vi "New Input Gallery.vi"(8 "Error In":errorcluster) -> (0 "Error Out":errorcluster, 3 "New Input Gallery":refnum<class "QWidget.lvclass">)   [LabVIEW 2014]
doc: "Dynamically assembles a widget that contains a variety of input widgets (text editors, combo boxes, and spinboxes). These widgets are grouped within group boxes.\n\nThe caller must manually make the returned widget visible.\n\n\nCopyright (c) 2019 Sze Howe Koh.\nThis code is licensed under the MIT license."
uses:
  <vilib>/addons/LQ/Qt Widgets/QWidget/QWidget.lvclass
  <vilib>/addons/LQ/Qt Widgets/QBoxLayout/Direction.ctl
  <vilib>/addons/LQ/Qt Widgets/QLineEdit/EchoMode.ctl
  <vilib>/addons/LQ/Qt Widgets/QLineEdit/setPlaceholderText.vi
  <vilib>/addons/LQ/Qt Widgets/QLineEdit/setEchoMode.vi
  <vilib>/addons/LQ/Qt Widgets/QTextEdit/QTextEdit.lvclass
  <vilib>/addons/LQ/Qt Widgets/QLineEdit/QLineEdit.lvclass
  <vilib>/addons/LQ/Qt Widgets/QGroupBox/QGroupBox.lvclass
  <vilib>/addons/LQ/Qt Widgets/QBoxLayout/QBoxLayout.lvclass
  <vilib>/addons/LQ/Qt Widgets/QComboBox/QComboBox.lvclass
  <vilib>/addons/LQ/Qt Widgets/QSpinBox/QSpinBox.lvclass
  <vilib>/addons/LQ/Qt Widgets/QDoubleSpinBox/QDoubleSpinBox.lvclass
  <vilib>/addons/LQ/Qt Widgets/QFontComboBox/QFontComboBox.lvclass
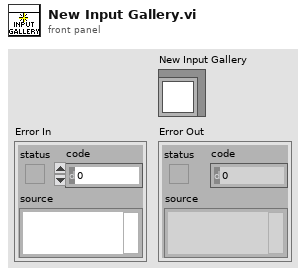
[diagram p1: front panel]
types:
  T1 = typedef "QLineEdit.lvclass/EchoMode.ctl" = i32
  T2 = typedef "QBoxLayout.lvclass/Direction.ctl" = i32
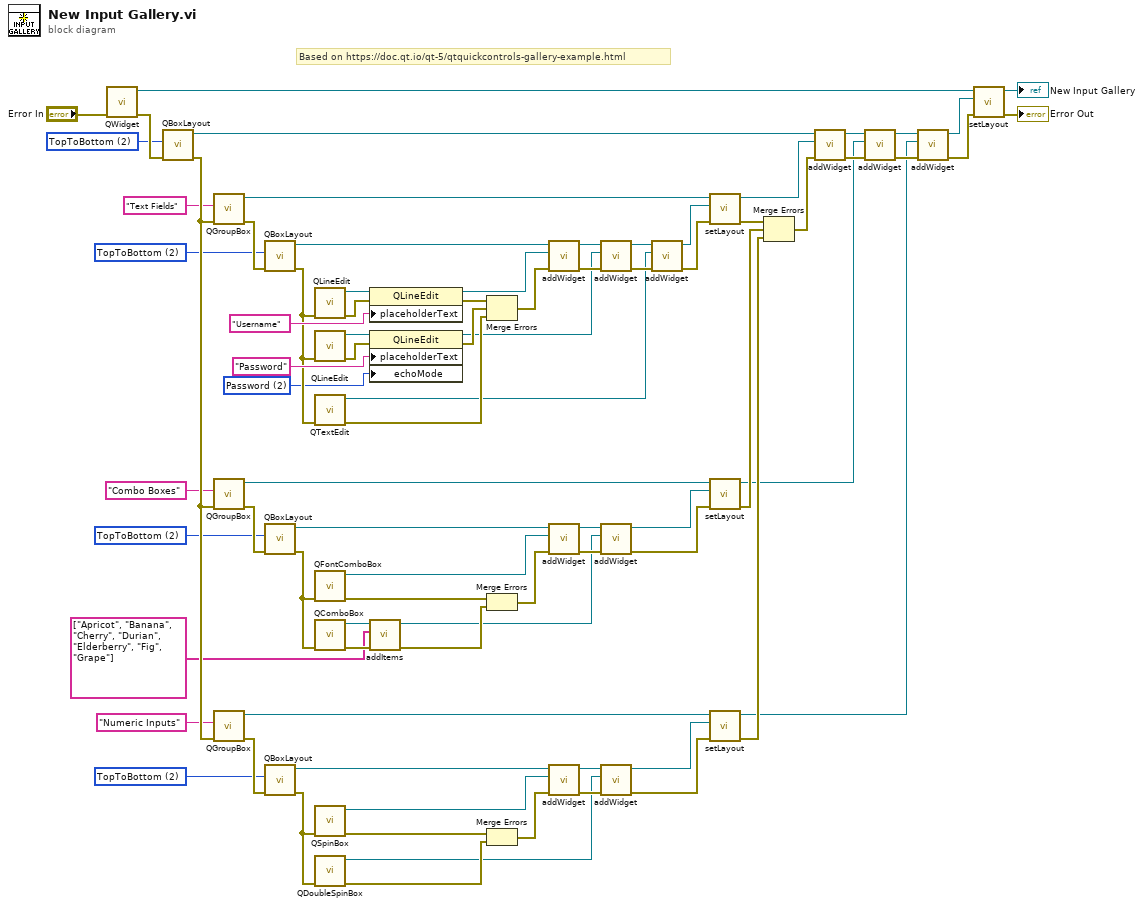
[diagram p0: block diagram]
diagram:
  w8 = T1 2 items=["Normal", "NoEcho", "Password", "PasswordEchoOnEdit"] ("echoMode")
  w48 = T2 2 items=["LeftToRight", "RightToLeft", "TopToBottom", "BottomToTop"] ("direction")
  w55 = T2 2 items=["LeftToRight", "RightToLeft", "TopToBottom", "BottomToTop"] ("direction")
  w56 = T2 2 items=["LeftToRight", "RightToLeft", "TopToBottom", "BottomToTop"] ("direction")
  w57 = T2 2 items=["LeftToRight", "RightToLeft", "TopToBottom", "BottomToTop"] ("direction")
  # "Based on https://doc.qt.io/qt-5/qtquickcontrols-gallery-example.html"
  n1 = call <vilib>:"QWidget.vi"("Error In"="Error In") -> ("Error Out"=w77:errorcluster, "New QWidget"=w58:refnum<class "QWidget.lvclass">)  [unwired: 9 in]
  n2 = call <vilib>:"QBoxLayout.vi"("Error In"=w77, "direction"=w56) -> ("Error Out"=w72:errorcluster, "New QBoxLayout"=w60:refnum<class "QBoxLayout.lvclass">)  [unwired: 8 in]
  n3 = call <vilib>:"QGroupBox.vi"("Error In"=w72, "title"="Text Fields") -> ("Error Out"=w78:errorcluster, "New QGroupBox"=w68:refnum<class "QGroupBox.lvclass">)  [unwired: 8 in]
  n4 = call <vilib>:"QGroupBox.vi"("Error In"=w72, "title"="Combo Boxes") -> ("Error Out"=w74:errorcluster, "New QGroupBox"=w61:refnum<class "QGroupBox.lvclass">)  [unwired: 8 in]
  n5 = call <vilib>:"QGroupBox.vi"("Error In"=w72, "title"="Numeric Inputs") -> ("Error Out"=w71:errorcluster, "New QGroupBox"=w41:refnum<class "QGroupBox.lvclass">)  [unwired: 8 in]
  n6 = call <vilib>:"QBoxLayout.vi"("Error In"=w78, "direction"=w57) -> ("Error Out"=w14:errorcluster, "New QBoxLayout"=w67:refnum<class "QBoxLayout.lvclass">)  [unwired: 8 in]
  n7 = call <vilib>:"QBoxLayout.vi"("Error In"=w74, "direction"=w55) -> ("Error Out"=w73:errorcluster, "New QBoxLayout"=w63:refnum<class "QBoxLayout.lvclass">)  [unwired: 8 in]
  n8 = call <vilib>:"QBoxLayout.vi"("Error In"=w71, "direction"=w48) -> ("Error Out"=w70:errorcluster, "New QBoxLayout"=w46:refnum<class "QBoxLayout.lvclass">)  [unwired: 8 in]
  n9 = call <vilib>:"QLineEdit.vi"("Error In"=w14) -> ("Error Out"=w18:errorcluster, "New QLineEdit"=w20:refnum<class "QLineEdit.lvclass">)  [unwired: 9 in]
  n10 = call <vilib>:"QLineEdit.vi"("Error In"=w14) -> ("Error Out"=w21:errorcluster, "New QLineEdit"=w23:refnum<class "QLineEdit.lvclass">)  [unwired: 9 in]
  n11 = call <vilib>:"QTextEdit.vi"("Error In"=w14) -> ("Error Out"=w80:errorcluster, "New QTextEdit"=w9:refnum<class "QTextEdit.lvclass">)  [unwired: 9 in]
  n12 = call <vilib>:"QFontComboBox.vi"("Error In"=w73) -> ("Error Out"=w53:errorcluster, "New QFontComboBox"=w26:refnum<class "QFontComboBox.lvclass">)  [unwired: 9 in]
  n13 = call <vilib>:"QComboBox.vi"("Error In"=w73) -> ("Error Out"=w4:errorcluster, "New QComboBox"=w5:refnum<class "QComboBox.lvclass">)  [unwired: 9 in]
  n14 = call <vilib>:"QSpinBox.vi"("Error In"=w70) -> ("Error Out"=w45:errorcluster, "New QSpinBox"=w28:refnum<class "QSpinBox.lvclass">)  [unwired: 9 in]
  n15 = call <vilib>:"QDoubleSpinBox.vi"("Error In"=w70) -> ("Error Out"=w44:errorcluster, "New QDoubleSpinBox"=w27:refnum<class "QDoubleSpinBox.lvclass">)  [unwired: 9 in]
  n16 = property class="QLineEdit"(reference=w20, error in=w18, "placeholderText"="Username" ("text")) -> (reference out=w19:refnum<class "QLineEdit.lvclass">, error out=w17:errorcluster)
  n17 = property class="QLineEdit"(reference=w23, error in=w21, "placeholderText"="Password" ("text"), "echoMode"=w8) -> (reference out=w22:refnum<class "QLineEdit.lvclass">, error out=w79:errorcluster)
  n18 = call <vilib>:"addItems.vi"("Error In"=w4, "texts"=string[] ["Apricot", "Banana", "Cherry", "Durian", "Elderberry", "Fig", "Grape"], "QComboBox In"=w5) -> ("Error Out"=w3:errorcluster, "QComboBox Out"=w2:refnum<class "QComboBox.lvclass">)  [unwired: 7 in]
  n19 = Merge Errors(w17, w79, w80) -> (w54:errorcluster)
  n20 = Merge Errors(w53, w3) -> (w52:errorcluster)
  n21 = Merge Errors(w45, w44) -> (w43:errorcluster)
  n22 = call <vilib>:"addWidget.vi"("Error In"=w54, "widget"=w19, "QBoxLayout In"=w67) -> ("Error Out"=w76:errorcluster, "QBoxLayout Out"=w66:refnum<class "QBoxLayout.lvclass">)  [unwired: 7 in]
  n23 = call <vilib>:"addWidget.vi"("Error In"=w52, "widget"=w26, "QBoxLayout In"=w63) -> ("Error Out"=w75:errorcluster, "QBoxLayout Out"=w62:refnum<class "QBoxLayout.lvclass">)  [unwired: 7 in]
  n24 = call <vilib>:"addWidget.vi"("Error In"=w43, "widget"=w28, "QBoxLayout In"=w46) -> ("Error Out"=w42:errorcluster, "QBoxLayout Out"=w47:refnum<class "QBoxLayout.lvclass">)  [unwired: 7 in]
  n25 = call <vilib>:"addWidget.vi"("Error In"=w76, "widget"=w22, "QBoxLayout In"=w66) -> ("Error Out"=w11:errorcluster, "QBoxLayout Out"=w13:refnum<class "QBoxLayout.lvclass">)  [unwired: 7 in]
  n26 = call <vilib>:"addWidget.vi"("Error In"=w75, "widget"=w2, "QBoxLayout In"=w62) -> ("Error Out"=w29:errorcluster, "QBoxLayout Out"=w30:refnum<class "QBoxLayout.lvclass">)  [unwired: 7 in]
  n27 = call <vilib>:"addWidget.vi"("Error In"=w42, "widget"=w27, "QBoxLayout In"=w47) -> ("Error Out"=w6:errorcluster, "QBoxLayout Out"=w7:refnum<class "QBoxLayout.lvclass">)  [unwired: 7 in]
  n28 = call <vilib>:"addWidget.vi"("Error In"=w11, "widget"=w9, "QBoxLayout In"=w13) -> ("Error Out"=w10:errorcluster, "QBoxLayout Out"=w12:refnum<class "QBoxLayout.lvclass">)  [unwired: 7 in]
  n29 = call <vilib>:"setLayout.vi"("Error In"=w10, "layout"=w12, "QWidget In"=w68) -> ("Error Out"=w35:errorcluster, "QWidget Out"=w36:refnum<class "QGroupBox.lvclass">)  [unwired: 7 in]
  n30 = call <vilib>:"setLayout.vi"("Error In"=w29, "layout"=w30, "QWidget In"=w61) -> ("Error Out"=w25:errorcluster, "QWidget Out"=w24:refnum<class "QGroupBox.lvclass">)  [unwired: 7 in]
  n31 = call <vilib>:"setLayout.vi"("Error In"=w6, "layout"=w7, "QWidget In"=w41) -> ("Error Out"=w69:errorcluster, "QWidget Out"=w34:refnum<class "QGroupBox.lvclass">)  [unwired: 7 in]
  n32 = Merge Errors(w35, w25, w69) -> (w51:errorcluster)
  n33 = call <vilib>:"addWidget.vi"("Error In"=w51, "widget"=w36, "QBoxLayout In"=w60) -> ("Error Out"=w50:errorcluster, "QBoxLayout Out"=w59:refnum<class "QBoxLayout.lvclass">)  [unwired: 7 in]
  n34 = call <vilib>:"addWidget.vi"("Error In"=w50, "widget"=w24, "QBoxLayout In"=w59) -> ("Error Out"=w38:errorcluster, "QBoxLayout Out"=w40:refnum<class "QBoxLayout.lvclass">)  [unwired: 7 in]
  n35 = call <vilib>:"addWidget.vi"("Error In"=w38, "widget"=w34, "QBoxLayout In"=w40) -> ("Error Out"=w37:errorcluster, "QBoxLayout Out"=w39:refnum<class "QBoxLayout.lvclass">)  [unwired: 7 in]
  n36 = call <vilib>:"setLayout.vi"("Error In"=w37, "layout"=w39, "QWidget In"=w58) -> ("Error Out"=→"Error Out":errorcluster, "QWidget Out"=→"New Input Gallery":refnum<class "QWidget.lvclass">)  [unwired: 7 in]
